vi "A 铜环有无结果分析.vi"(8 "Tbl引用句柄":refnum<vi>, 11 "Histogram (Histogram 1)":u32[][](array[numeric])) -> ()   [LabVIEW 2017]
panel:
  out "0, 1":i16
  out "x > y?":bool
  out "元素索引":i32
  out "子数组":u32[](array[numeric])
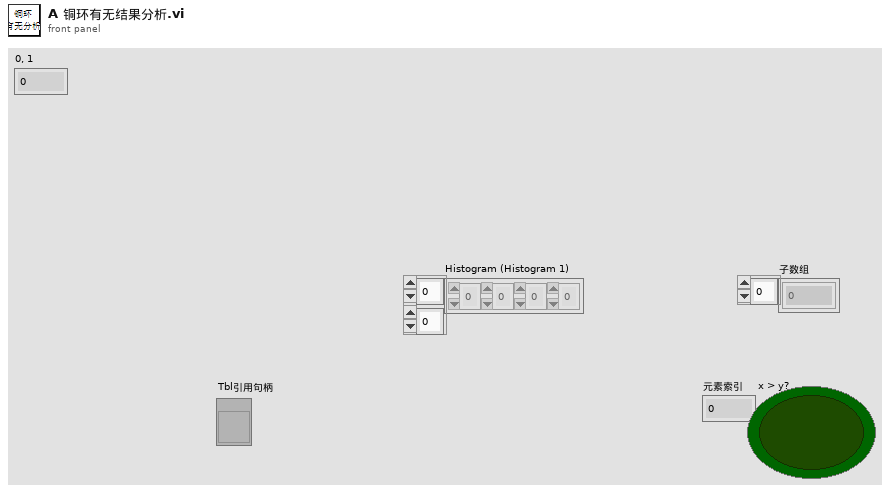
[diagram p1: front panel]
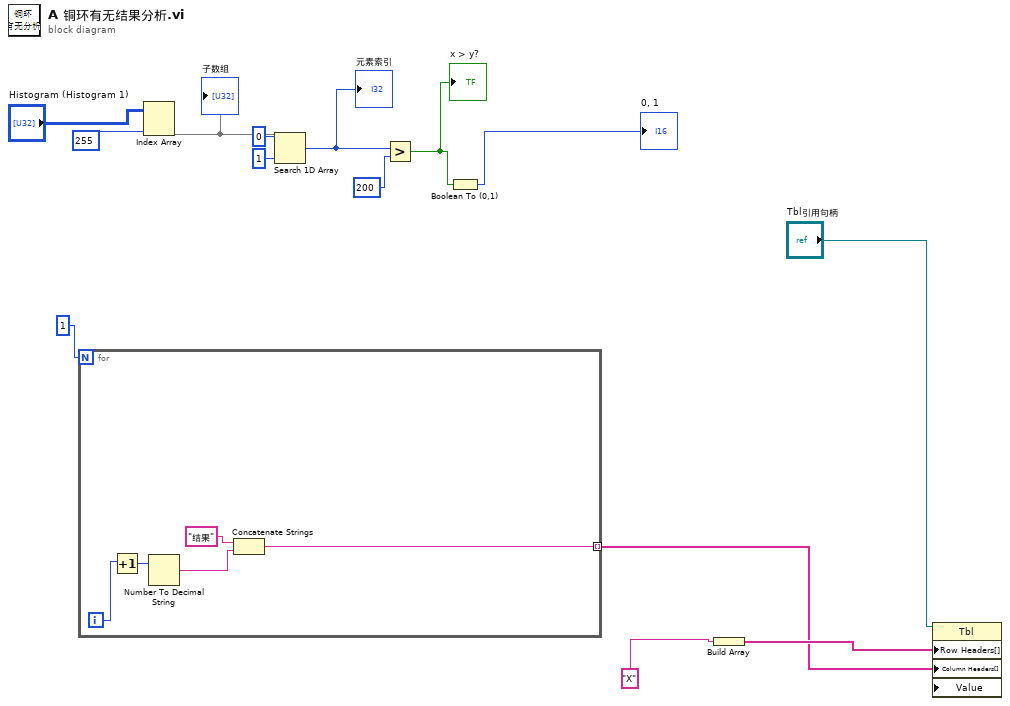
[diagram p0: block diagram]
diagram:
  n1 = for {
    N: 1 -> [_]
    tunnel: [w17] -> w10 mode=indexing
    i -> [w16]
    n2 = Increment(x=w16) -> (x+1=w15:i32)
    n3 = Number To Decimal String(number=w15) -> (decimal integer string=w18:string)  [unwired: 1 in]
    n4 = Concatenate Strings("结果", w18) -> (w17:string)
  }
  n5 = Index Array(array="Histogram (Histogram 1)", index (row)=255 ("索引 (行)")) -> (element=w7:u32[])  [unwired: 1 in]
  "子数组" <- w7
  n6 = Search 1D Array(1D array=w7, element=u32 0 ("元素"), start index (0)=1 ("开始索引(0)")) -> (index of element=w5:i32)
  "元素索引" <- w5
  n7 = Greater?(x=w5, y=200) -> (0:w2:bool)
  "x > y?" <- w2
  n8 = Boolean To (0,1)(Boolean=w2) -> (0, 1=→"0, 1":i16)
  n9 = Build Array("X") -> (w12:string[])
  n10 = property class="Tbl" props=["Row Headers[]", "Column Headers[]", "Value"](reference="Tbl引用句柄", "Row Headers[]"=w12, "Column Headers[]"=w10) -> ()  [unwired: 2 in, 2 out]
